vi "光源通訊_FGV.vi"(7 "通訊_action":T1, 8 "error in (no error)":errorcluster, 9 "亮度":u8, 10 "通道":u8=1 min=1 max=4, 11 "VISA resource name":refnum<visa-resource-name>) -> (0 "error out":errorcluster, 3 "回應值":string)   [LabVIEW 2015]
uses:
  <vilib>/Instr/_visa.llb/VISA Configure Serial Port (Instr).vi
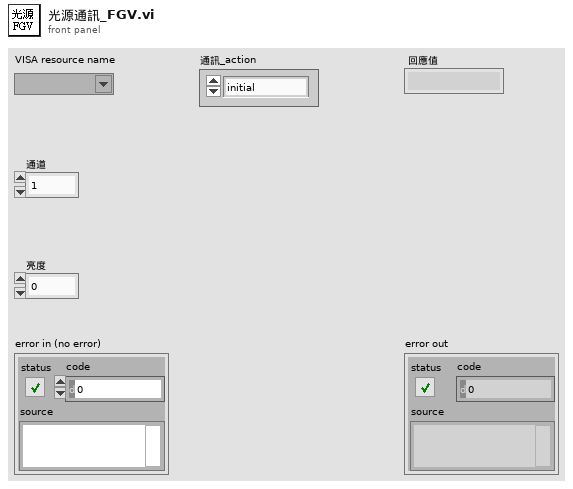
[diagram p1: front panel]
types:
  T1 = typedef "光源通訊_action_control.ctl" = enum16{"initial", "開啟光源", "關閉光源", "close"}
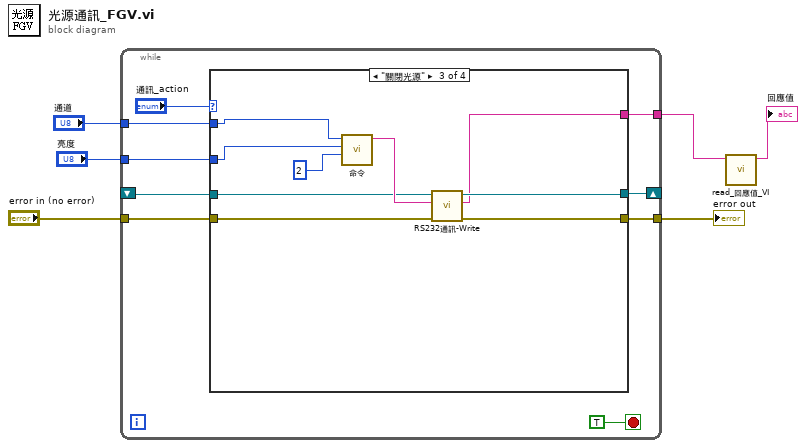
[diagram p0: block diagram]
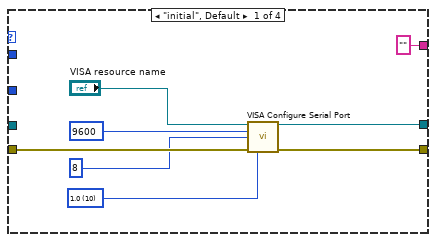
[diagram p2: hidden frame]
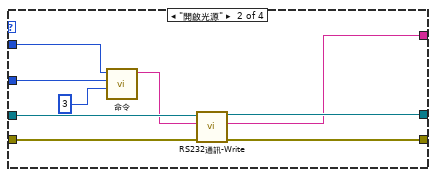
[diagram p3: hidden frame]
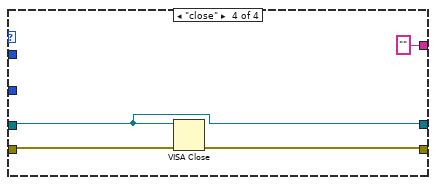
[diagram p4: hidden frame]
diagram:
  n1 = while {
    shift-right: [w11] -> _
    shift-left: _ -> [w10]
    tunnel: "error in (no error)" -> [w13]
    tunnel: [w12] -> w5
    tunnel: "亮度" -> [w9]
    tunnel: [w8] -> w3
    tunnel: "通道" -> [w7]
    stop <- TRUE stop-if-true
    n2 = case shown="\"關閉光源\"" "通訊_action" {
      tunnel: w13 -> [w23 w32 w39 w45]
      tunnel: [w22 w31 w38 w44] -> w12
      tunnel: [w21 w30 w37 w43] -> w11
      tunnel: w10 -> [_ w29 w36 w43]
      tunnel: w9 -> [_ w26 w34 _]
      tunnel: ["" ("read buffer") w25 w35 "" ("read buffer")] -> w8
      tunnel: w7 -> [_ w24 w33 _]
      frame "initial", Default {
        w16 = u16 10 items=["1.0"=10, "1.5"=15, "2.0"=20] ("stop bits (10: 1 bit)")
        n3 = call-poly "VISA Configure Serial Port"("VISA resource name"="VISA resource name", "baud rate (9600)"=u32 9600, "data bits (8)"=u16 8, "error in (no error)"=w23, "stop bits (10: 1 bit)"=w16) -> ("VISA resource name out"=w21:refnum<visa-resource-name>, "error out"=w22:errorcluster)  [unwired: 9 in]
      }
      frame "開啟光源" {
        n4 = call "命令.vi"("命令值"=u8 3, "亮度"=w26, "通道"=w24) -> ("concatenated string 2"=w28:string)  [unwired: 8 in]
        n5 = call "RS232通訊-Write.vi"("error in (no error)"=w32, "string"=w28, "VISA Refnum in"=w29) -> ("error out"=w31:errorcluster, "read buffer"=w25:string, "VISA resource name out"=w30:refnum<visa-resource-name>)  [unwired: 6 in]
      }
      frame "關閉光源" {
        n6 = call "命令.vi"("命令值"=u8 2, "亮度"=w34, "通道"=w33) -> ("concatenated string 2"=w41:string)  [unwired: 8 in]
        n7 = call "RS232通訊-Write.vi"("error in (no error)"=w39, "string"=w41, "VISA Refnum in"=w36) -> ("error out"=w38:errorcluster, "read buffer"=w35:string, "VISA resource name out"=w37:refnum<visa-resource-name>)  [unwired: 6 in]
      }
      frame "close" {
        n8 = VISA Close(VISA resource name=w43, error in (no error)=w45) -> (error out=w44:errorcluster)
      }
    }
  }
  "error out" <- w5
  n9 = call "read_回應值_VI.vi"("read buffer"=w3) -> ("回應值"=→"回應值":string)  [unwired: 10 in]
